vi "Position of Padding Zero for FFT.vi"() -> ()   [LabVIEW 2013]
uses:
  <vilib>/Analysis/2dsp.llb/Real FFT.vi
  <vilib>/Analysis/NI_AALPro.lvlib
panel:
  out "Waveform Graph 2":dbl[][](graph)
  out "Waveform Graph":dbl[][](graph)
  in  "Array 1":dbl[](array[numeric])
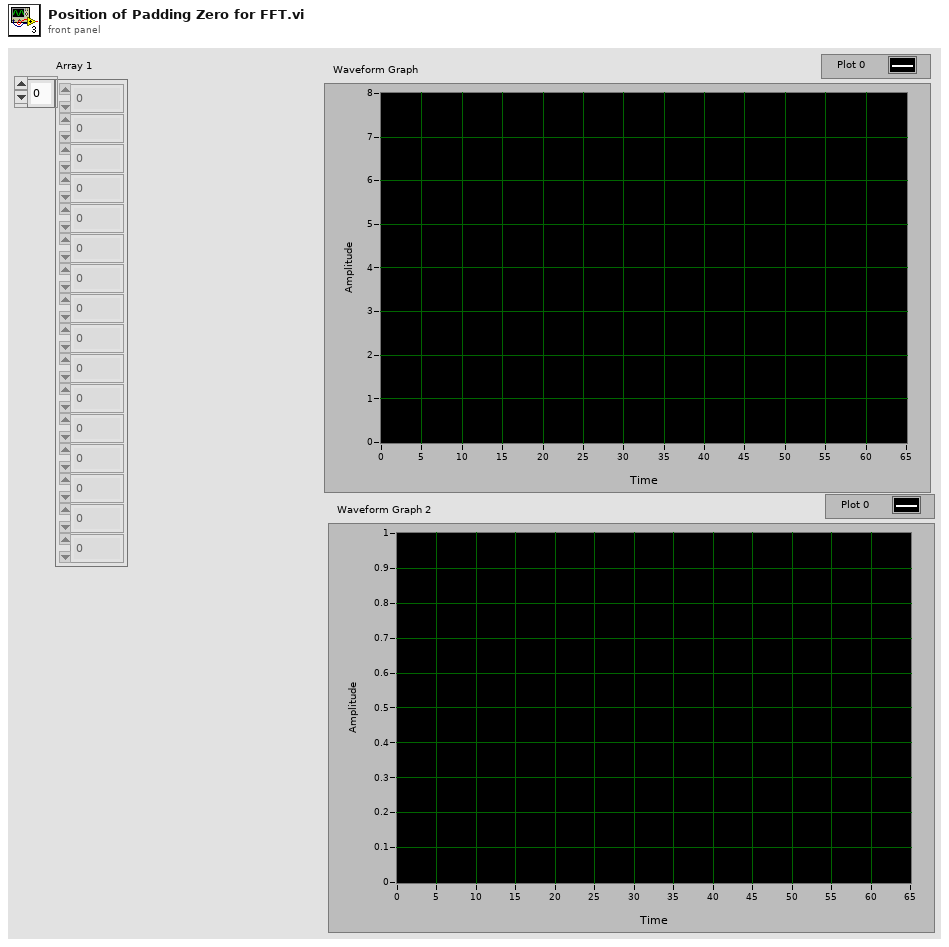
[diagram p1: front panel]
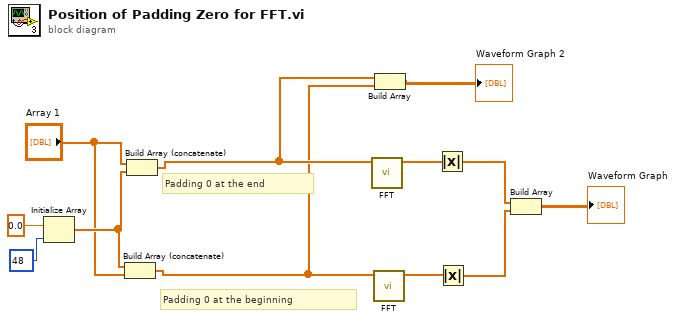
[diagram p0: block diagram]
diagram:
  # "Padding 0 at the beginning"
  # "Padding 0 at the end"
  n1 = Initialize Array(0.0 ("element"), 48 ("dimension size")) -> (w5:dbl[])
  n2 = Build Array (concatenate)(w5, "Array 1") -> (w2:dbl[])
  n3 = Build Array (concatenate)("Array 1", w5) -> (w3:dbl[])
  n4 = call-poly <vilib>:"FFT.vi"("X"=w3) -> ("FFT {X}"=w12:cdb[])  [unwired: 9 in, 1 out]
  n5 = call-poly <vilib>:"FFT.vi"("X"=w2) -> ("FFT {X}"=w11:cdb[])  [unwired: 9 in, 1 out]
  n6 = Build Array(w3, w2) -> (→"Waveform Graph 2":dbl[][])
  n7 = Absolute Value(x=w12) -> (abs(x)=w10:dbl[])
  n8 = Absolute Value(x=w11) -> (abs(x)=w9:dbl[])
  n9 = Build Array(w10, w9) -> (→"Waveform Graph":dbl[][])
